vi "07 - Channel metadata.vi"() -> ()   [LabVIEW 2020]
uses:
  client/client.lvlib
panel:
  out "name equal":bool
  out "description equal":bool
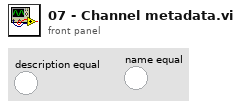
[diagram p1: front panel]
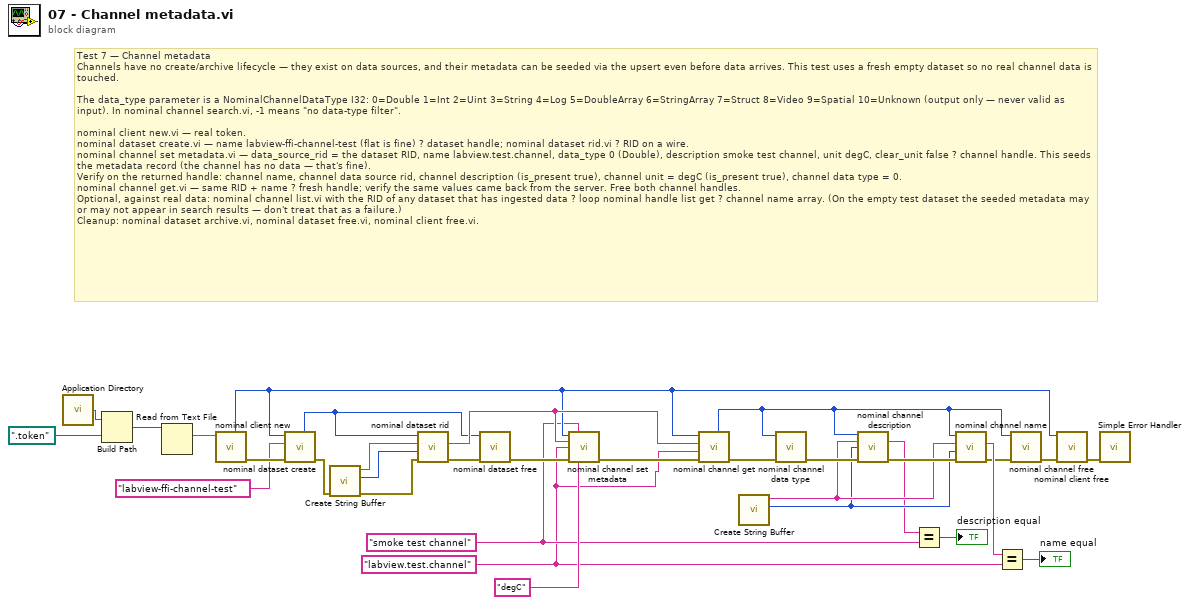
[diagram p0: block diagram]
diagram:
  w3 = "smoke test channel" ("name")
  w1 = "labview.test.channel" ("name")
  # "Test 7 — Channel metadata\nChannels have no create/archive lifecycle — they exist on data sources, and their metadata can be seeded via the upsert even before data arrives. This test uses a fresh empty dataset so no real channel data is touched.\n\nThe data_type parameter is a NominalChannelDataType I32: 0=Double 1=Int 2=Uint 3=String 4=Log 5=DoubleArray 6=StringArray 7=Struct 8=Video 9=Spatial 10=Unknown (output only — never valid as input). In nominal channel search.vi, -1 means \"no data-type filter\".\n\nnominal client new.vi — real token.\nnominal dataset create.vi — name labview-ffi-channel-test (flat is fine) ? dataset handle; nominal dataset rid.vi ? RID on a wire.\nnominal channel set metadata.vi — data_source_rid = the dataset RID, name labview.test.channel, data_type 0 (Double), description smoke test channel, unit degC, clear_unit false ? channel handle. This seeds the metadata record (the channel has no data — that's fine).\nVerify on the returned handle: channel name, channel data source rid, channel description (is_present true), channel unit = degC (is_present true), channel data type = 0.\nnominal channel get.vi — same RID + name ? fresh handle; verify the same values came back from the server. Free both channel handles.\nOptional, against real data: nominal channel list.vi with the RID of any dataset that has ingested data ? loop nominal handle list get ? channel name array. (On the empty test dataset the seeded metadata may or may not appear in search results — don't treat that as a failure.)\nCleanup: nominal dataset archive.vi, nominal dataset free.vi, nominal client free.vi."
  n1 = call <vilib>:"Application Directory.vi"() -> ("Application Directory"=w31:path)
  n2 = Build Path(base path=w31, name or relative path=path ".token") -> (appended path=w29:path)
  n3 = Read from Text File(file (use dialog)=w29) -> (text=w5:string)  [unwired: 3 in, 3 out]
  n4 = call "nominal client new.vi"("token"=w5) -> ("error out"=w28:errorcluster, "out_client out"=w4:i32)  [unwired: 8 in, 1 out]
  n5 = call "nominal dataset create.vi"("error in (no error)"=w28, "name"="labview-ffi-channel-test", "client"=w4) -> ("error out"=w23:errorcluster, "out_dataset out"=w8:i32)  [unwired: 6 in, 1 out]
  n6 = call "Create String Buffer.vi"("error in"=w23) -> ("error out"=w24:errorcluster, "dub Buffer Size"=w25:i32, "String Buffer"=w26:string)  [unwired: 8 in]
  n7 = call "nominal dataset rid.vi"("error in (no error)"=w24, "cap"=w25, "buf"=w26, "dataset"=w8) -> ("error out"=w7:errorcluster, "buf out"=w21:string)  [unwired: 4 in, 2 out]
  n8 = call "nominal dataset free.vi"("error in (no error)"=w7, "dataset"=w8) -> ("error out"=w6:errorcluster)  [unwired: 8 in, 1 out]
  n9 = call "nominal channel set metadata.vi"("client"=w4, "description"=w3, "data_source_rid"=w21, "name"=w1, "error in (no error)"=w6, "unit"="degC" ("name")) -> ("error out"=w2:errorcluster)  [unwired: 7 in, 2 out]
  n10 = call "nominal channel get.vi"("error in (no error)"=w2, "name"=w1, "data_source_rid"=w21, "client"=w4) -> ("error out"=w18:errorcluster, "out_channel out"=w11:i32)  [unwired: 5 in, 1 out]
  n11 = call "Create String Buffer.vi"() -> ("dub Buffer Size"=w16:i32, "String Buffer"=w17:string)  [unwired: 9 in, 1 out]
  n12 = call "nominal channel data type.vi"("error in (no error)"=w18, "channel"=w11) -> ("error out"=w19:errorcluster)  [unwired: 7 in, 2 out]
  n13 = call "nominal channel description.vi"("channel"=w11, "buf"=w17, "cap"=w16, "error in (no error)"=w19) -> ("buf out"=w15:string, "error out"=w20:errorcluster)  [unwired: 7 in, 3 out]
  n14 = Equal?(x=w15, y=w3) -> (x = y?=→"description equal":bool)
  n15 = call "nominal channel name.vi"("error in (no error)"=w20, "cap"=w16, "buf"=w17, "channel"=w11) -> ("error out"=w10:errorcluster, "buf out"=w14:string)  [unwired: 4 in, 2 out]
  n16 = Equal?(x=w14, y=w1) -> (x = y?=→"name equal":bool)
  n17 = call "nominal channel free.vi"("error in (no error)"=w10, "channel"=w11) -> ("error out"=w9:errorcluster)  [unwired: 8 in, 1 out]
  n18 = call "nominal client free.vi"("error in (no error)"=w9, "client"=w4) -> ("error out"=w32:errorcluster)  [unwired: 8 in, 1 out]
  n19 = call <vilib>:"Simple Error Handler.vi"("error in (no error)"=w32) -> ()  [unwired: 4 in, 5 out]
